vi "ADI_IMU_ADIS16448_Loop.vi"(8 "error in":errorcluster, 11 "ADI IMU DevRef":T1={"DevStatus"={"status"=FALSE, "code"=0, "source"=""}, "Handle"=0, "SPI Bus"=enum."SPI On-Board, CS0", "Device Found"=FALSE, "Device Ready"=FALSE, "Yaw Axis"=enum."Z", "AHRS Algorithm"=enum."Complementary", "Serial"=0, "Lot ID 2"=0, "Lot ID 1"=0, "Bytes Per Sample"=0, "Calibrate On Open?"=FALSE}) -> (1 "Device Found":bool)   [LabVIEW 2018, in "ADIS16448_IMU.lvlib"]
doc: "Periodically reads the ADI MXP IMU valuse and makes data available for use elsewhere in your robot project. Place this block within PeriodicTasks.vi outside any loops."
uses:
  ADIS16448_IMU.lvlib
  ADI_IMU_ADIS16448_IMUDevRef.ctl
  <vilib>/Rock Robotics/SystemInterfaces/spilib/spi_bus.ctl
  <vilib>/Rock Robotics/Network Tables/NT Write Number.vi
panel:
  in  "Main Name":string
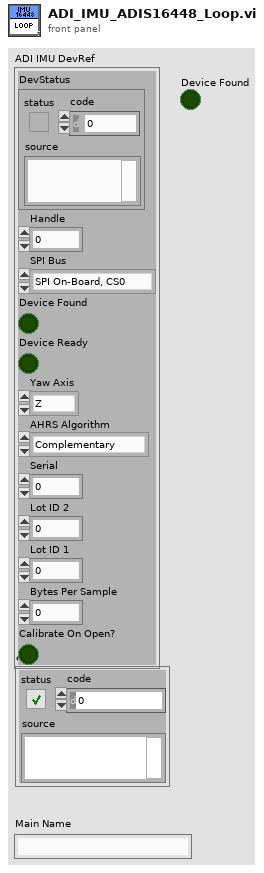
[diagram p1: front panel]
types:
  T1 = typedef "ADIS16448_IMU.lvlib/ADI_IMU_ADIS16448_IMUDevRef.ctl" = cluster{"DevStatus":errorcluster, "Handle":i32, "SPI Bus":T2, "Device Found":bool, "Device Ready":bool, "Yaw Axis":enum16{"X", "Y", "Z"}, "AHRS Algorithm":enum16{"Complementary", "Madgwick"}, "Serial":u16, "Lot ID 2":u16, "Lot ID 1":u16, "Bytes Per Sample":u16, "Calibrate On Open?":bool}
  T2 = typedef "spi_bus.ctl" = enum16{"SPI On-Board, CS0", "SPI On-Board, CS1", "SPI On-Board, CS2", "SPI On-Board, CS3", "SPI MXP", "Invalid"}
  T3 = cluster{"X Angle":dbl, "Y Angle":dbl, "Z Angle":dbl}
  T4 = enum32{"Bad", "Idle", "Run top level", "Running"}
  T5 = cluster{"X Gyro":dbl, "Y Gyro":dbl, "Z Gyro":dbl, "X Accel":dbl, "Y Accel":dbl, "Z Accel":dbl, "X Mag":dbl, "Y Mag":dbl, "Z Mag":dbl, "Pressure":dbl, "Temp":dbl}
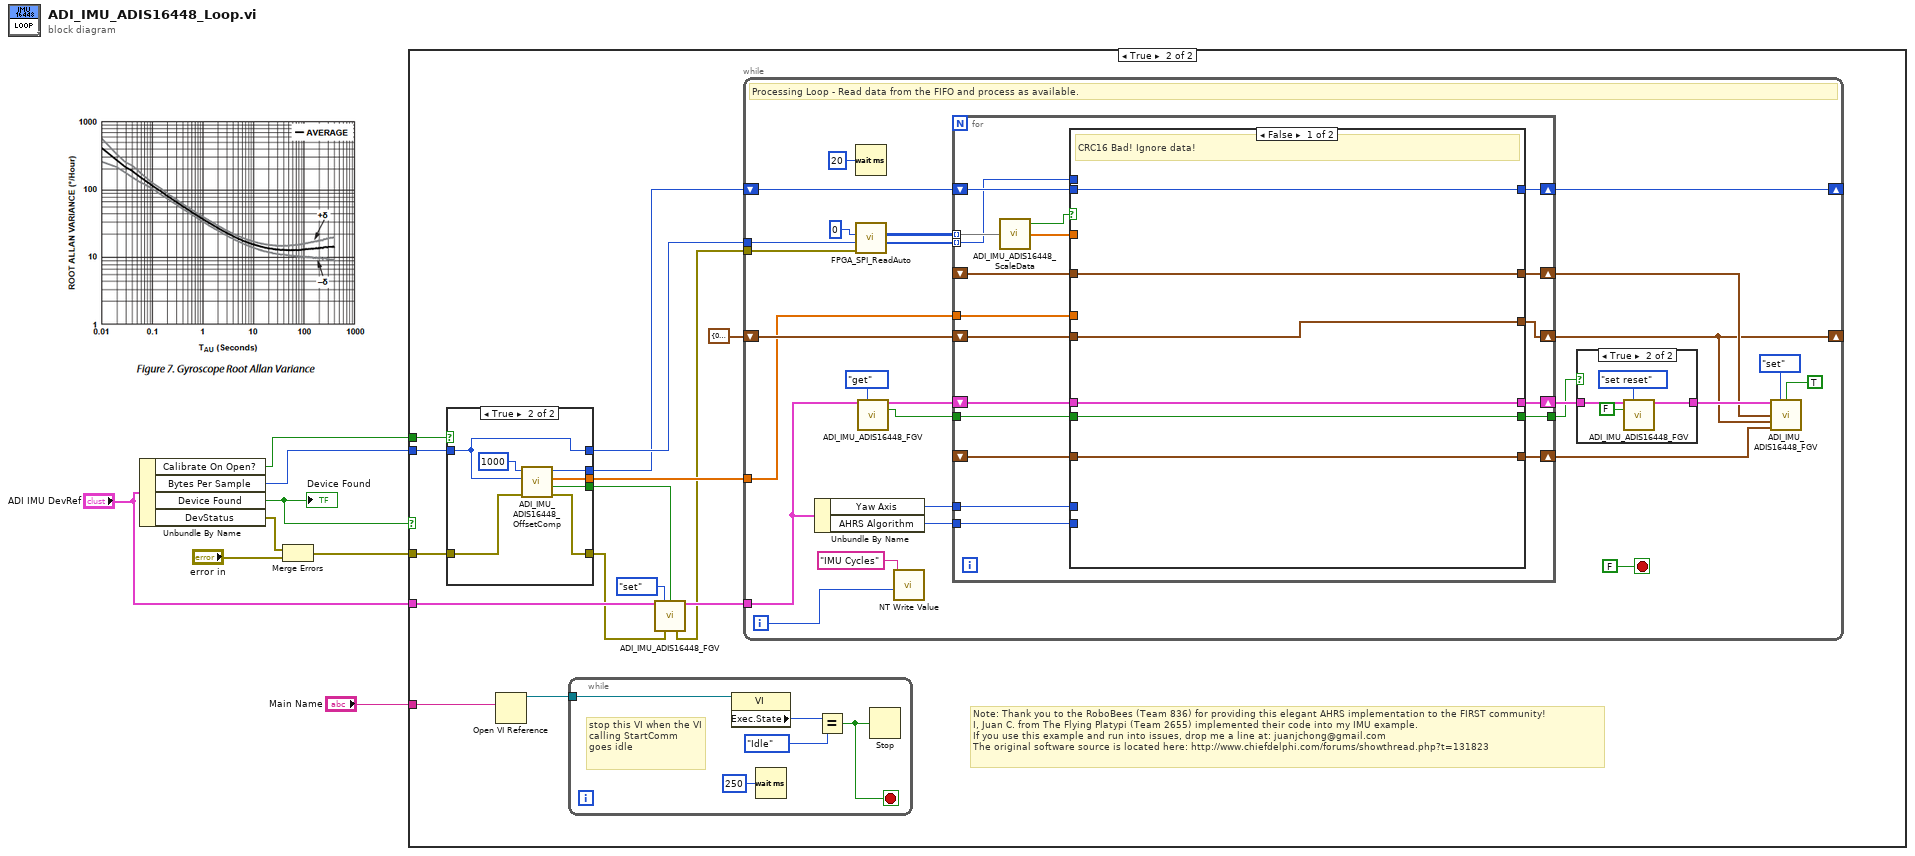
[diagram p0: block diagram]
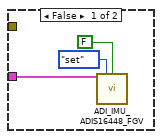
[diagram p2: hidden frame]
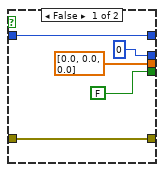
[diagram p3: hidden frame]
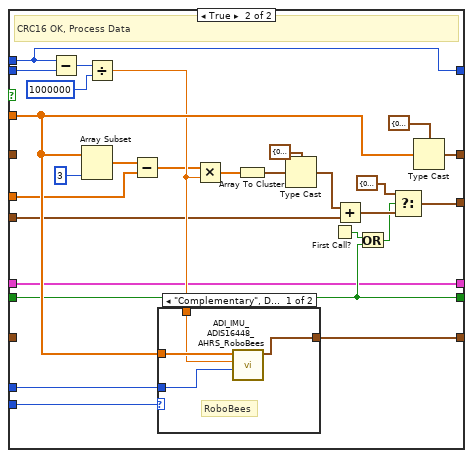
[diagram p4: hidden frame]
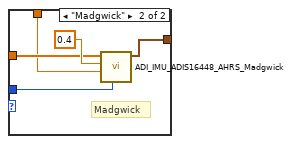
[diagram p5: hidden frame]
diagram:
  n1 = Unbundle By Name("ADI IMU DevRef") -> ("Calibrate On Open?"=w1:bool, "Bytes Per Sample"=w3:u16, "Device Found"=w5:bool, "DevStatus"=w6:errorcluster)
  "Device Found" <- w5
  n2 = Merge Errors(w6, "error in") -> (w2:errorcluster)
  n3 = case shown="True" w5 {
    tunnel: "Main Name" -> [_ w25]
    tunnel: "ADI IMU DevRef" -> [w10 w24]
    tunnel: w3 -> [_ w18]
    tunnel: w2 -> [_ w19]
    tunnel: w1 -> [_ w20]
    frame False {
      n4 = call "ADI_IMU_ADIS16448_FGV.vi"("ADI IMU DevRef"=w10, "Operation"=enum16{"set", "get", "set reset"}."set", "Sensor Ready?"=FALSE) -> ()  [unwired: 6 in, 7 out]
    }
    frame True {
      # "Note: Thank you to the RoboBees (Team 836) for providing this elegant AHRS implementation to the FIRST community!\nI, Juan C. from The Flying Platypi (Team 2655) implemented their code into my IMU example.\nIf you use this example and run into issues, drop me a line at: juanjchong@gmail.com\nThe original software source is located here: http://www.chiefdelphi.com/forums/showthread.php?t=131823"
      n5 = case shown="True" w20 {
        tunnel: w19 -> [w30 w38]
        tunnel: [w30 w37] -> w13
        tunnel: w18 -> [w29 w34]
        tunnel: [FALSE ("Sensor Ready?") w35] -> w17
        tunnel: [w29 w34] -> w16
        tunnel: [dbl[] [0.0, 0.0, 0.0] ("Offsets") w33] -> w15
        tunnel: [u32 0 ("Timestamp") w32] -> w14
        frame False {
        }
        frame True {
          n6 = call "ADI_IMU_ADIS16448_OffsetComp.vi"("error in"=w38, "Bytes per Sample"=w34, "n Samples"=u32 1000) -> ("error out"=w37:errorcluster, "Sensor Ready?"=w35:bool, "Offsets"=w33:dbl[], "Timestamp"=w32:u32)  [unwired: 3 in]
        }
      }
      n7 = Open VI Reference(vi path=w25) -> (vi reference=w26:refnum<vi>)  [unwired: 1 in, 5 out]
      n8 = while {
        tunnel: w26 -> [w40]
        stop <- w39 stop-if-true
        # "stop this VI when the VI calling StartComm goes idle"
        n9 = property class="VI"(reference=w40) -> ("Exec.State"=w42:T4)  [unwired: 1 in, 2 out]
        n10 = Wait (ms)(milliseconds to wait=u32 250) -> ()  [unwired: 1 out]
        n11 = Equal?(x=w42, y=T4."Idle" ("Execution:State")) -> (x = y?=w39:bool)
        n12 = Stop(stop? (T)=w39) -> ()
      }
      n13 = call "ADI_IMU_ADIS16448_FGV.vi"("ADI IMU DevRef"=w24, "Operation"=enum16{"set", "get", "set reset"}."set", "Sensor Ready?"=w17, "error in"=w13) -> ("ADI IMU DevRef Out"=w23:T1, "error out"=w12:errorcluster)  [unwired: 5 in, 5 out]
      n14 = while {
        tunnel: w23 -> [w53]
        tunnel: w16 -> [w60]
        tunnel: w12 -> [w59]
        shift-right: [w51] -> _
        shift-left: T3 {"X Angle"=0.0, "Y Angle"=0.0, "Z Angle"=0.0} ("IMU Angles") -> [w57]
        tunnel: w15 -> [w49]
        shift-right: [w46] -> _
        shift-left: w14 -> [w48]
        i -> [w44]
        stop <- FALSE stop-if-true
        # "Processing Loop - Read data from the FIFO and process as available."
        n15 = Unbundle By Name(w53) -> ("Yaw Axis"=w69:enum16{"X", "Y", "Z"}, "AHRS Algorithm"=w68:enum16{"Complementary", "Madgwick"})
        n16 = Wait (ms)(milliseconds to wait=u32 20) -> ()  [unwired: 1 out]
        n17 = call <vilib>:"FPGA_SPI_ReadAuto.vi"("error in (no error)"=w59, "Bytes per Sample"=w60, "Samples to Read"=u32 0) -> ("Timestamps"=w47:u32[], "Data"=w56:u8[][])  [unwired: 6 in, 1 out]
        n18 = call "ADI_IMU_ADIS16448_FGV.vi"("ADI IMU DevRef"=w53, "Operation"=enum16{"set", "get", "set reset"}."get") -> ("ADI IMU DevRef Out"=w54:T1, "Reset Out"=w52:bool)  [unwired: 7 in, 5 out]
        n19 = call-poly <vilib>:"NT Write Value.vi"("Numeric"=w44, "Name"="IMU Cycles") -> ()  [unwired: 9 in, 1 out]
        n20 = for {
          tunnel: w69 -> [w87]
          tunnel: w68 -> [w86]
          tunnel: [w77] -> w63
          tunnel: w49 -> [w82]
          shift-right: [w88] -> w51
          shift-left: w57 -> [w89]
          shift-right: [w71] -> w65
          shift-left: w54 -> [w72]
          tunnel: w56 -> [w81] mode=indexing
          tunnel: w52 -> [w78]
          shift-right: [w85] -> w62
          shift-left: _ -> [w79]
          shift-right: [w75] -> w46
          shift-left: w48 -> [w76]
          shift-right: [w83] -> w58
          shift-left: _ -> [w74]
          tunnel: w47 -> [w73] mode=indexing
          n21 = call "ADI_IMU_ADIS16448_ScaleData.vi"("Received Data"=w81) -> ("Data Array"=w84:dbl[], "Data Good?"=w80:bool)  [unwired: 3 in]
          n22 = case shown="False" w80 {
            tunnel: w89 -> [w95 w101]
            tunnel: [w95 w100] -> w88
            tunnel: w87 -> [_ w122]
            tunnel: w86 -> [_ w121]
            tunnel: [w94 w115] -> w85
            tunnel: w84 -> [_ w114]
            tunnel: [w92 w113] -> w83
            tunnel: w82 -> [_ w104]
            tunnel: w79 -> [w94 _]
            tunnel: [w93 w97] -> w77
            tunnel: w78 -> [w93 w97]
            tunnel: w76 -> [w91 w112]
            tunnel: [w91 w111] -> w75
            tunnel: w74 -> [w92 _]
            tunnel: w73 -> [_ w111]
            tunnel: w72 -> [w90 w96]
            tunnel: [w90 w96] -> w71
            frame False {
              # "CRC16 Bad! Ignore data!"
            }
            frame True {
              # "CRC16 OK, Process Data"
              n23 = Subtract(x=w111, y=w112) -> (x-y=w110:u32)
              n24 = Array Subset(array=w114, length=3) -> (w105:dbl[])  [unwired: 1 in]
              n25 = Divide(x=w110, y=u32 1000000) -> (x/y=w108:dbl)
              n26 = Subtract(x=w105, y=w104) -> (x-y=w103:dbl[])
              n27 = case shown="\"Complementary\", Default" w121 {
                tunnel: w114 -> [w126 w130]
                tunnel: w122 -> [w125 w129]
                tunnel: [w124 w128] -> w115
                tunnel: w108 -> [w123 w127]
                frame "Complementary", Default {
                  # "RoboBees"
                  n28 = call "ADI_IMU_ADIS16448_AHRS_RoboBees.vi"("Yaw Axis"=w125, "Delta t"=w123, "IMU Rates"=w126) -> ("Output"=w124:cluster{"Pitch":dbl, "Roll":dbl, "Yaw":dbl})  [unwired: 4 in, 3 out]
                }
                frame "Madgwick" {
                  # "Madgwick"
                  n29 = call "ADI_IMU_ADIS16448_AHRS_Madgwick.vi"("Yaw Axis"=w129, "delta t"=w127, "Beta"=0.4, "Data"=w130) -> ("Output"=w128:cluster{"Pitch":dbl, "Roll":dbl, "Yaw":dbl})  [unwired: 7 in]
                }
              }
              n30 = Multiply(x=w103, y=w108) -> (x*y=w107:dbl[])
              n31 = Array To Cluster(array=w107) -> (cluster=w106:cluster{"[0]":dbl, "[1]":dbl, "[2]":dbl})
              n32 = Type Cast(type=T3 {"X Angle"=0.0, "Y Angle"=0.0, "Z Angle"=0.0} ("IMU Angles"), x=w106) -> (*(type *) &x=w118:T3)
              n33 = First Call?() -> (First Call?: T/F=w98:bool)
              n34 = Add(x=w118, y=w101) -> (x+y=w102:T3)
              n35 = Or(x=w98, y=w97) -> (x .or. y?=w99:bool)
              n36 = Select(t=T3 {"X Angle"=0.0, "Y Angle"=0.0, "Z Angle"=0.0} ("IMU Angles"), s=w99, f=w102) -> (s? t:f=w100:T3)
              n37 = Type Cast(type=T5 {"X Gyro"=0.0, "Y Gyro"=0.0, "Z Gyro"=0.0, "X Accel"=0.0, "Y Accel"=0.0, "Z Accel"=0.0, "X Mag"=0.0, "Y Mag"=0.0, "Z Mag"=0.0, "Pressure"=0.0, "Temp"=0.0} ("IMU Data"), x=w114) -> (*(type *) &x=w113:T5)
            }
          }
        }
        n38 = case shown="True" w63 {
          tunnel: [w132 w135] -> w66
          tunnel: w65 -> [w132 w134]
          frame False {
          }
          frame True {
            n39 = call "ADI_IMU_ADIS16448_FGV.vi"("ADI IMU DevRef"=w134, "Operation"=enum16{"set", "get", "set reset"}."set reset", "Reset"=FALSE) -> ("ADI IMU DevRef Out"=w135:T1)  [unwired: 6 in, 6 out]
          }
        }
        n40 = call "ADI_IMU_ADIS16448_FGV.vi"("ADI IMU DevRef"=w66, "Operation"=enum16{"set", "get", "set reset"}."set", "Sensor Ready?"=TRUE, "IMU Data"=w58, "IMU Angles"=w51, "IMU AHRS"=w62) -> ()  [unwired: 3 in, 7 out]
      }
    }
  }
